vi "HalfSpeed.vi"(9 "R In":dbl, 10 "Y In":dbl, 11 "X In":dbl) -> (1 "R Out":dbl, 2 "Y Out":dbl, 3 "X Out":dbl)   [LabVIEW 2014]
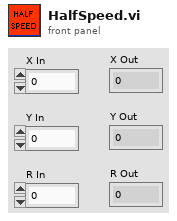
[diagram p1: front panel]
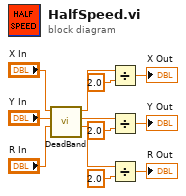
[diagram p0: block diagram]
diagram:
  n1 = call "DeadBand.vi"("R In"="R In", "Y In"="Y In", "X In"="X In") -> ("R Out"=w3:dbl, "Y Out"=w2:dbl, "X Out"=w1:dbl)  [unwired: 6 in]
  n2 = Divide(x=w1, y=2.0) -> (x/y=→"X Out":dbl)
  n3 = Divide(x=w2, y=2.0) -> (x/y=→"Y Out":dbl)
  n4 = Divide(x=w3, y=2.0) -> (x/y=→"R Out":dbl)
